vi "Bernoulli Moments.vi"(9 "p":dbl=0.2) -> (0 "error":i32, 2 "variance":dbl=0.8, 3 "mean":dbl=0.2)   [LabVIEW 2018, in "NI_Gmath.lvlib"]
doc: "Returns the expected mean and variance of the random variate X, where X describes the selected distribution type. You must manually select the polymorphic instance to use."
uses:
  NI_Gmath.lvlib
  st_error_code.ctl
panel:
  # "Bernoulli Moments"
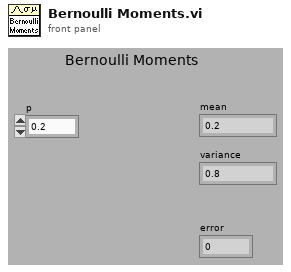
[diagram p1: front panel]
types:
  T1 = typedef "NI_Gmath.lvlib/st_error_code.ctl" = i32
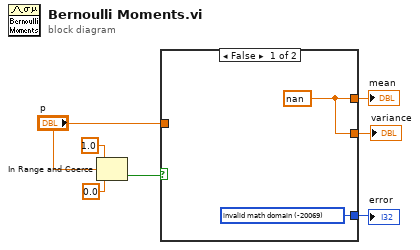
[diagram p0: block diagram]
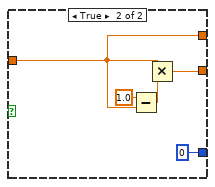
[diagram p2: hidden frame]
diagram:
  n1 = In Range and Coerce(upper limit=1.0, x="p", lower limit=0.0) -> (In Range?=w5:bool)  [unwired: 1 out]
  n2 = case shown="False" w5 {
    tunnel: [w9 w11] -> w4
    tunnel: [w9 w10] -> w3
    tunnel: [w8 0 ("error")] -> w2
    tunnel: "p" -> [_ w11]
    frame False {
      w8 = T1 -20069 items=["invalid math domain"=-20069, "Fourier interpolation size m >= n"=-20070, "empty array"=-20003] ("stat interp error code")
      w9 = nan
    }
    frame True {
      n3 = Subtract(x=1.0, y=w11) -> (x-y=w12:dbl)
      n4 = Multiply(x=w11, y=w12) -> (x*y=w10:dbl)
    }
  }
  "error" <- w2
  "mean" <- w4
  "variance" <- w3
